vi "Write to File.vi"(8 "error in":errorcluster, 10 "LogRecord in":refnum<class "LogRecord.lvclass">, 11 "File Ref":refnum<file>) -> (0 "error out":errorcluster)   [LabVIEW 2020, in "hse-logger.lvlib" / "FileHandler.lvclass"]
doc: "Write the information from the logRecord to a file. The format is static.\n\n____\nHAMPEL SOFTWARE ENGINEERING v2.0.6 (2021-04-15 11:38)"
uses:
  FileHandler.lvclass
  LogRecord/LogRecord.lvclass
  LogRecord/LogRecord.lvclass/LogRecord.ctl
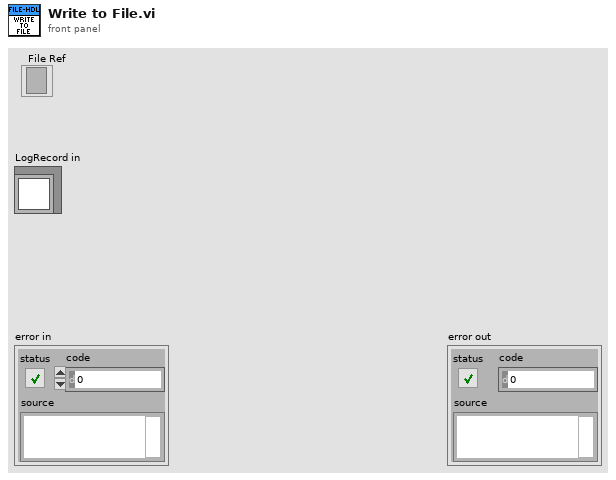
[diagram p1: front panel]
types:
  T1 = typedef "hse-logger.lvlib/LogLevel.ctl" = enum16{"DEBUG", "INFO", "WARNING", "ERROR", "CRITICAL"}
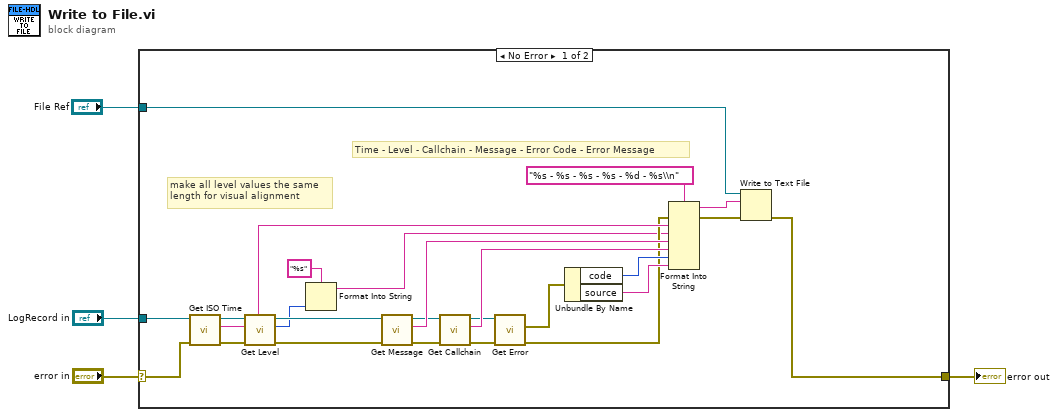
[diagram p0: block diagram]
diagram:
  n1 = case shown="No Error" "error in" {
    selector: "error in" -> [w12 w30]
    tunnel: "LogRecord in" -> [w29 _]
    tunnel: "File Ref" -> [w8 _]
    tunnel: [w11 w30] -> w1
    frame No Error {
      # "make all level values the same \nlength for visual alignment"
      # "Time - Level - Callchain - Message - Error Code - Error Message"
      n2 = call "Get ISO Time.vi"("error in"=w12, "LogRecord in"=w29) -> ("error out"=w16:errorcluster, "ISO Time"=w23:string, "LogRecord out"=w15:refnum<class "LogRecord.lvclass">)  [unwired: 7 in]
      n3 = call "Get Level.vi"("error in"=w16, "LogRecord in"=w15) -> ("error out"=w18:errorcluster, "Level"=w7:T1, "LogRecord out"=w17:refnum<class "LogRecord.lvclass">)  [unwired: 7 in]
      n4 = Format Into String(format string="%s", w7) -> (resulting string=w5:string)  [unwired: 2 in, 1 out]
      n5 = call "Get Message.vi"("error in"=w18, "LogRecord in"=w17) -> ("error out"=w19:errorcluster, "Message"=w24:string, "LogRecord out"=w20:refnum<class "LogRecord.lvclass">)  [unwired: 7 in]
      n6 = call "Get Callchain.vi"("error in"=w19, "LogRecord in"=w20) -> ("error out"=w22:errorcluster, "Callchain"=w25:string, "LogRecord out"=w21:refnum<class "LogRecord.lvclass">)  [unwired: 7 in]
      n7 = call "Get Error.vi"("error in"=w22, "LogRecord in"=w21) -> ("error out"=w13:errorcluster, "Error"=w26:errorcluster)  [unwired: 7 in, 1 out]
      n8 = Unbundle By Name(w26) -> ("code"=w27:i32, "source"=w28:string)
      n9 = Format Into String(format string="%s - %s - %s - %s - %d - %s\\n", error in=w13, w23, w5, w24, w25, w27, w28) -> (resulting string=w9:string, error out=w10:errorcluster)  [unwired: 1 in]
      n10 = Write to Text File(file (use dialog)=w8, text=w9, error in=w10) -> (error out=w11:errorcluster)  [unwired: 1 in, 2 out]
    }
    frame Error {
    }
  }
  "error out" <- w1
